vi "Drive_Sensor_To_Angle.vi"(1 "Position (Raw Sensor Units)":dbl=4549.0) -> (0 "Numeric":dbl=39.814453125)   [LabVIEW 2019]
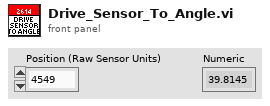
[diagram p1: front panel]
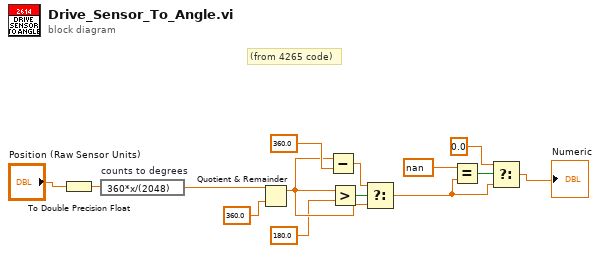
[diagram p0: block diagram]
diagram:
  # "(from 4265 code)"
  n1 = To Double Precision Float(number="Position (Raw Sensor Units)") -> (double precision float=w13:dbl)
  n2 = expression code="360*x/(2048)" "counts to degrees"(w13) -> (w14:dbl)
  n3 = Quotient & Remainder(x=w14, y=360.0) -> (x-y*floor(x/y)=w10:dbl)  [unwired: 1 out]
  n4 = Subtract(x=w10, y=360.0) -> (x-y=w11:dbl)
  n5 = Greater?(x=w10, y=180.0) -> (0:w9:bool)
  n6 = Select(t=w11, s=w9, f=w10) -> (s? t:f=w4:dbl)
  n7 = Equal?(x=nan, y=w4) -> (x = y?=w5:bool)
  n8 = Select(t=0.0, s=w5, f=w4) -> (s? t:f=→"Numeric":dbl)
